vi "Enbl-Dsbl-Ctrl's.vi"(0 "Quick-GUI-Update in":refnum<class "Quick-GUI-Update.lvclass">, 2 "Ctrl-Label":string[](array[string]), 11 "error in (no error)":errorcluster, 13 "Enbl-Dsbl":i32=3) -> (4 "Quick-GUI-Update out":refnum<class "Quick-GUI-Update.lvclass">, 15 "error out":errorcluster)   [LabVIEW 2020, in "Quick-GUI-Update.lvclass"]
doc: "<b>Enable Disable</b>\n1---><b>Enable</b> control's based on the Ctrl-Label input.\n2---><b>Disable</b> control's based on the Ctrl-Label input.\n3---><b>Diable and Grayed Out</b> control's based on the Ctrl-Label input.\n4---><b>Enable All</b> control's present in the front panel."
uses:
  Quick-GUI-Update.lvclass
  Quick-GUI-Update.lvclass/Quick-GUI-Update.ctl
  Ctrl Reference's/Ctrl Reference's.lvclass
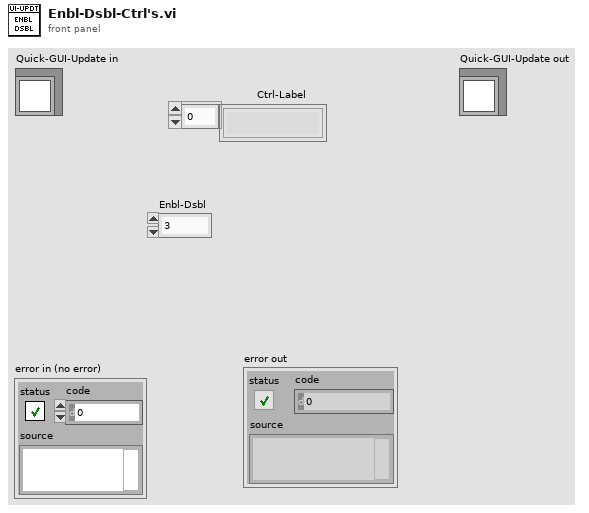
[diagram p1: front panel]
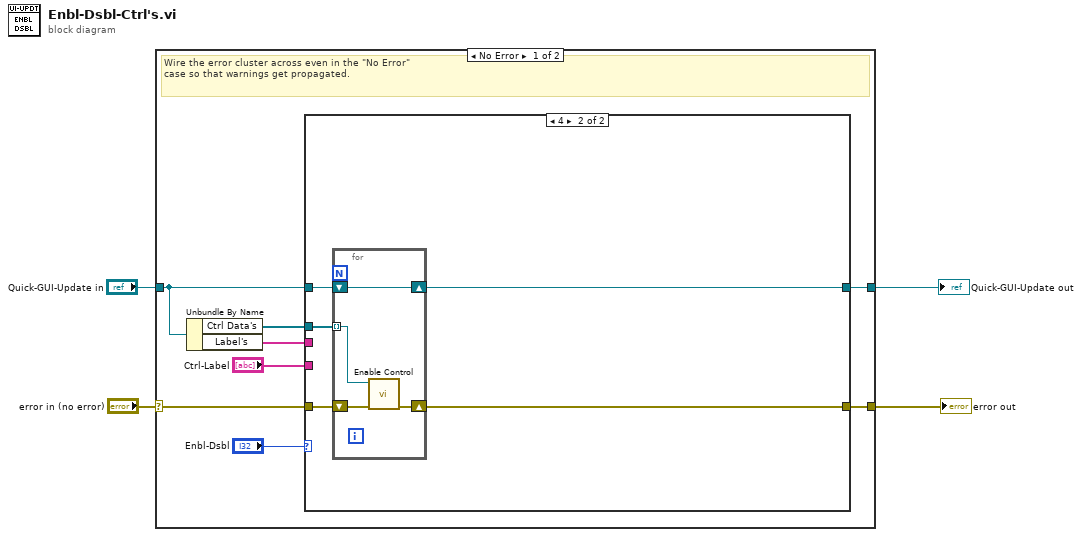
[diagram p0: block diagram]
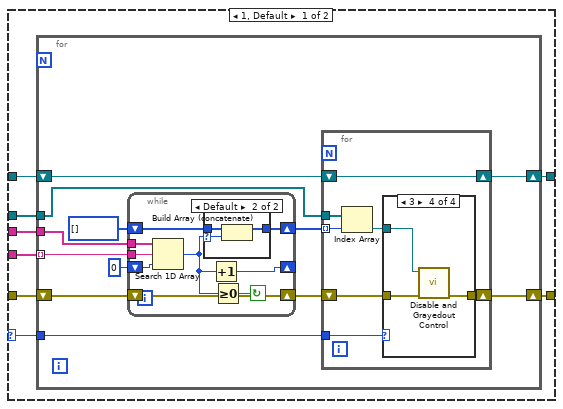
[diagram p2: hidden frame]
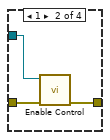
[diagram p4: hidden frame]
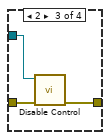
[diagram p5: hidden frame]
diagram:
  n1 = case shown="No Error" "error in (no error)" {
    selector: "error in (no error)" -> [w9 w72]
    tunnel: [w7 w73] -> w2
    tunnel: "Quick-GUI-Update in" -> [w8 w73]
    tunnel: [w6 w72] -> w1
    frame No Error {
      # "Wire the error cluster across even in the \"No Error\"\ncase so that warnings get propagated."
      n2 = Unbundle By Name(w8) -> ("Ctrl Data's"=w10:refnum<class "Ctrl Reference's.lvclass">[], "Label's"=w12:string[])
      n3 = case shown="4" "Enbl-Dsbl" {
        selector: "Enbl-Dsbl" -> [w13 _]
        tunnel: w12 -> [w20 _]
        tunnel: "Ctrl-Label" -> [w19 _]
        tunnel: w10 -> [w18 w67]
        tunnel: w9 -> [w17 w66]
        tunnel: w8 -> [w16 w65]
        tunnel: [w15 w64] -> w7
        tunnel: [w14 w63] -> w6
        frame 1, Default {
          n4 = for {
            tunnel: w20 -> [w26]
            tunnel: w19 -> [w25] mode=indexing
            tunnel: w18 -> [w32]
            tunnel: w13 -> [w30]
            shift-right: [w31] -> w14
            shift-left: w17 -> [w23]
            shift-right: [w21] -> w15
            shift-left: w16 -> [w22]
            n5 = while {
              shift-right: [w51] -> _
              shift-left: 0 ("Start Index (0)") -> [w58]
              shift-right: [w55] -> w27
              shift-left: i32[] [] ("Initial Elements") -> [w56]
              tunnel: w26 -> [w57]
              tunnel: w25 -> [w54]
              shift-right: [w50] -> w24
              shift-left: w23 -> [w50]
              stop <- w52 continue-if-true
              n6 = Search 1D Array(1D array=w57, element=w54, start index (0)=w58) -> (index of element=w53:i32)
              n7 = case shown="Default" w53 {
                selector: w53 -> [_ w62]
                tunnel: w56 -> [w59 w61]
                tunnel: [w59 w60] -> w55
                frame -1 {
                }
                frame Default {
                  n8 = Build Array (concatenate)(w61, w62) -> (w60:i32[])
                }
              }
              n9 = Increment(x=w53) -> (x+1=w51:i32)
              n10 = Greater Or Equal To 0?(x=w53) -> (x >= 0?=w52:bool)
            }
            n11 = for {
              shift-right: [w33] -> w31
              shift-left: w24 -> [w35]
              tunnel: w27 -> [w39] mode=indexing
              tunnel: w32 -> [w38]
              tunnel: w30 -> [w36]
              shift-right: [w37] -> w21
              shift-left: w22 -> [w37]
              n12 = Index Array(array=w38, index=w39) -> (element=w34:refnum<class "Ctrl Reference's.lvclass">)
              n13 = case shown="3" w36 {
                tunnel: w35 -> [w40 w43 w46 w49]
                tunnel: w34 -> [_ w42 w45 w48]
                tunnel: [w40 w41 w44 w47] -> w33
                frame 0, Default {
                }
                frame 1 {
                  n14 = call "Enable Control.vi"("error in (no error)"=w43, "Ctrl Reference's in"=w42) -> ("error out"=w41:errorcluster)  [unwired: 8 in, 1 out]
                }
                frame 2 {
                  n15 = call "Disable Control.vi"("error in (no error)"=w46, "Ctrl Reference's in"=w45) -> ("error out"=w44:errorcluster)  [unwired: 8 in, 1 out]
                }
                frame 3 {
                  n16 = call "Disable and Grayedout Control.vi"("error in (no error)"=w49, "Ctrl Reference's in"=w48) -> ("error out"=w47:errorcluster)  [unwired: 8 in, 1 out]
                }
              }
            }
          }
        }
        frame 4 {
          n17 = for {
            tunnel: w67 -> [w71] mode=indexing
            shift-right: [w70] -> w63
            shift-left: w66 -> [w69]
            shift-right: [w68] -> w64
            shift-left: w65 -> [w68]
            n18 = call "Enable Control.vi"("error in (no error)"=w69, "Ctrl Reference's in"=w71) -> ("error out"=w70:errorcluster)  [unwired: 8 in, 1 out]
          }
        }
      }
    }
    frame Error {
    }
  }
  "Quick-GUI-Update out" <- w2
  "error out" <- w1
